vi "keys.vi"() -> ()   [LabVIEW 2017]
panel:
  in  "Boolean 4":bool
  in  "Boolean 3":bool
  in  "Boolean 2":bool
  in  "Boolean":bool
  out "String":string
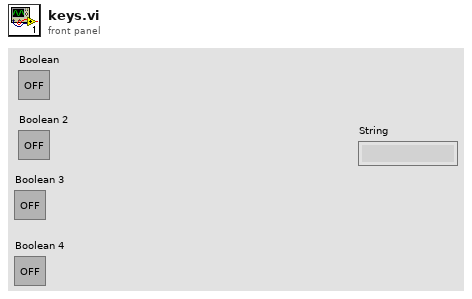
[diagram p1: front panel]
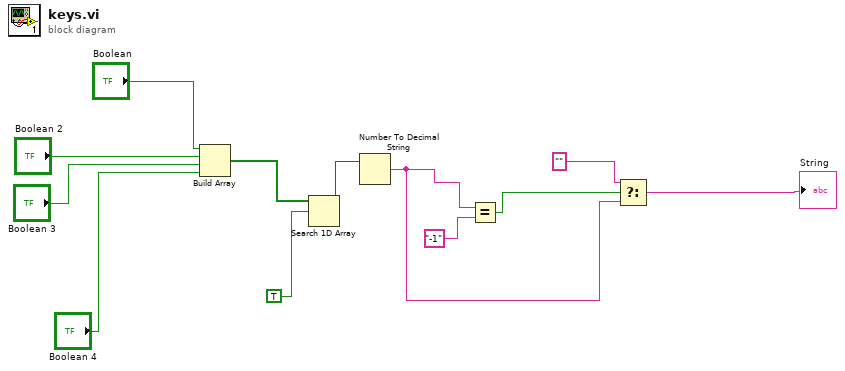
[diagram p0: block diagram]
diagram:
  n1 = Build Array("Boolean", "Boolean 2", "Boolean 3", "Boolean 4") -> (w12:bool[])
  n2 = Search 1D Array(1D array=w12, element=TRUE) -> (index of element=w10:i32)  [unwired: 1 in]
  n3 = Number To Decimal String(number=w10) -> (decimal integer string=w6:string)  [unwired: 1 in]
  n4 = Equal?(x=w6, y="-1") -> (x = y?=w8:bool)
  n5 = Select(t="" ("f"), s=w8, f=w6) -> (s? t:f=→"String":string)
